vi "Get_alloys_list.vi"(7 "LabVIEW Web Service Request":refnum<class "Web Request.lvclass">) -> (2 "Alloys_group_arr":T1(array[cluster]))   [LabVIEW 2020]
uses:
  <vilib>/wsapi/Web Request.lvclass
  <vilib>/Utility/file.llb/Read Delimited Spreadsheet (string).vi
panel:
  # "Use the Web Service Request input terminal to call the VIs on the Web Services palette. Do not remove it from the connector pane unless you don't need access to the palette."
  # "Each additional control wired to the connector pane will be available as an input in the URL. To include an indicator in terminal-mode output (the default setting), it must also be wired to the connector pane."
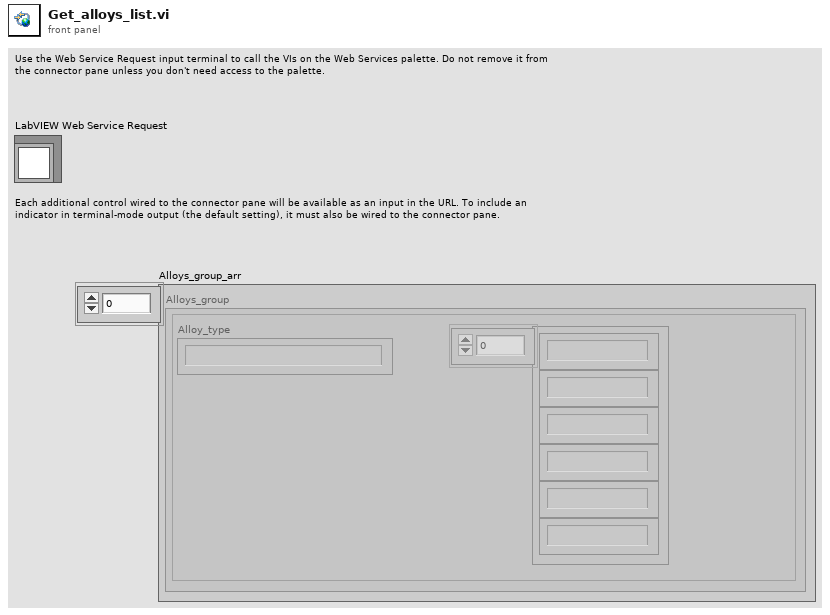
[diagram p1: front panel]
types:
  T1 = cluster{"Alloys":string[], "Alloy_type":string}[]
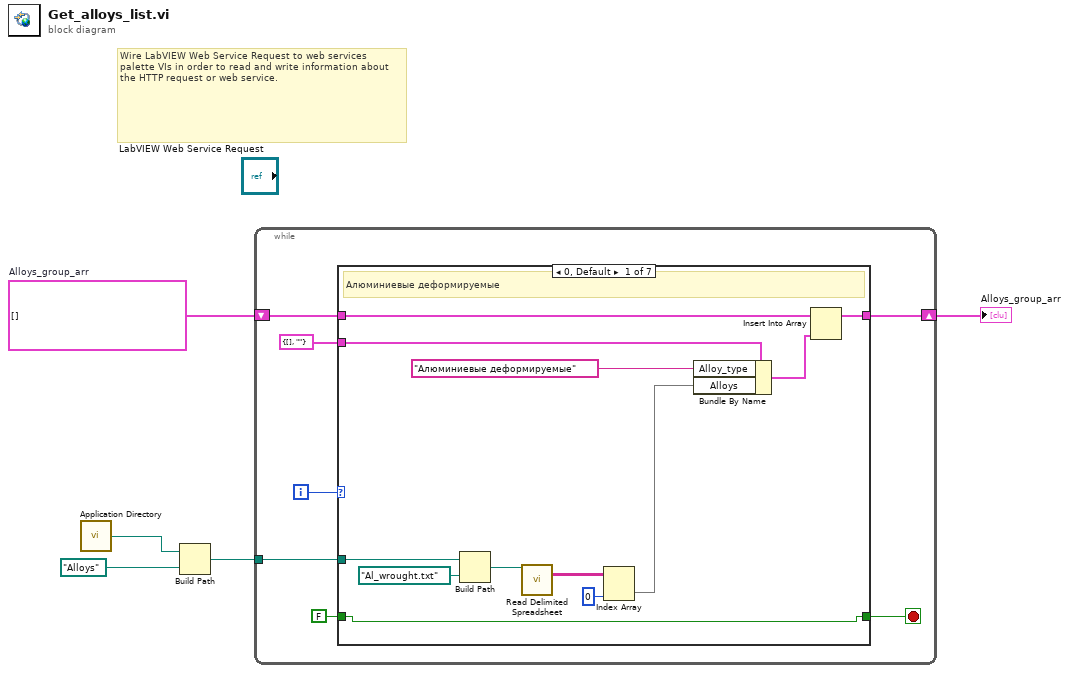
[diagram p0: block diagram]
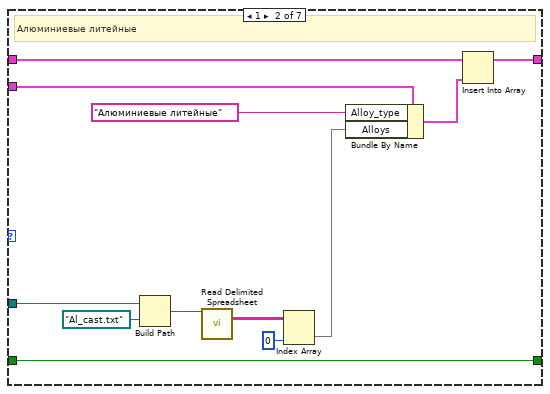
[diagram p2: hidden frame]
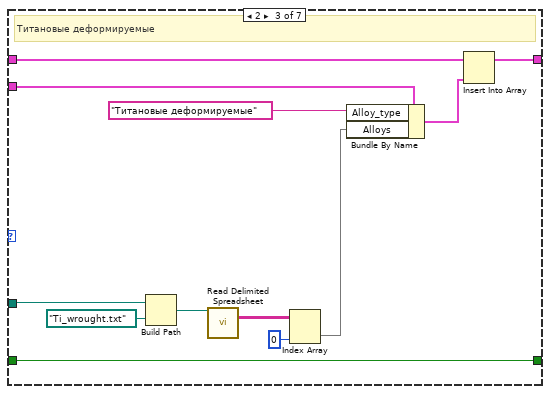
[diagram p3: hidden frame]
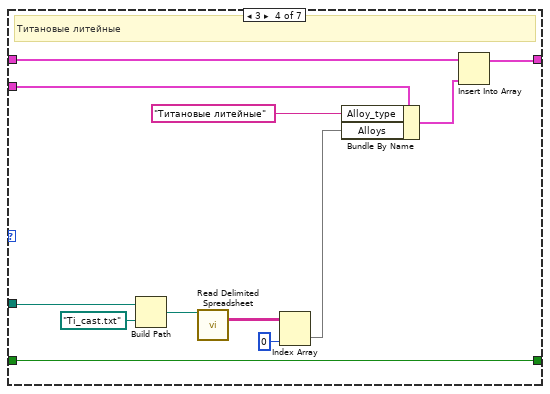
[diagram p4: hidden frame]
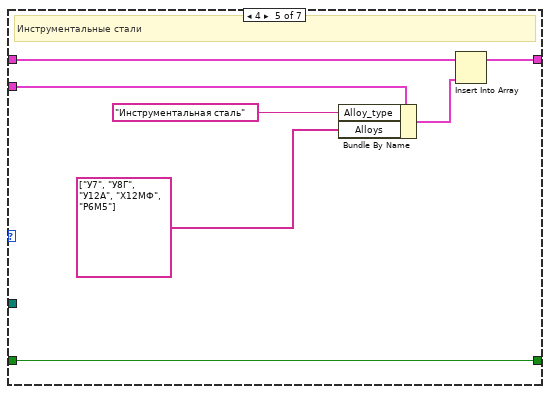
[diagram p5: hidden frame]
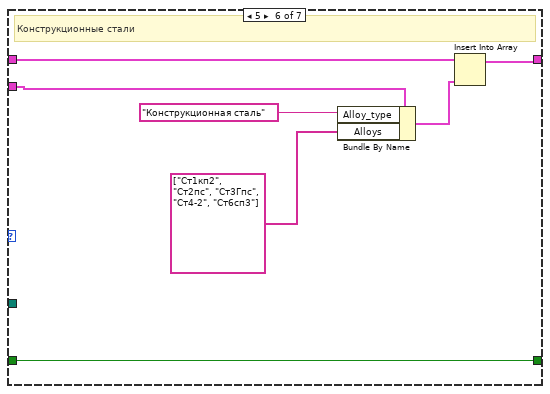
[diagram p6: hidden frame]
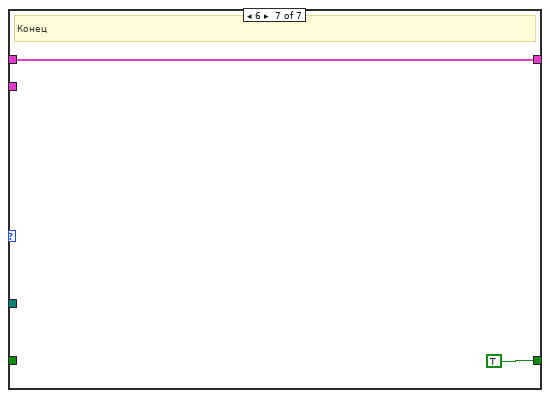
[diagram p7: hidden frame]
diagram:
  w5 = T1 []  # Alloys_group_arr
  # "Wire LabVIEW Web Service Request to web services palette VIs in order to read and write information about the HTTP request or web service."
  n1 = call <vilib>:"Application Directory.vi"() -> ("Application Directory"=w3:path)
  n2 = Build Path(base path=w3, name or relative path=path "Alloys") -> (appended path=w1:path)
  n3 = while {
    shift-right: [w10] -> w4
    shift-left: w5 -> [w9]
    tunnel: w1 -> [w7]
    i -> [w12]
    stop <- w11 stop-if-true
    n4 = case shown="0, Default" w12 {
      tunnel: [w17 w36 w48 w60 w67 w74 TRUE] -> w11
      tunnel: [w23 w34 w46 w58 w65 w71 w75] -> w10
      tunnel: w9 -> [w24 w33 w45 w57 w64 w72 w75]
      tunnel: cluster{"Alloys":string[], "Alloy_type":string} {"Alloys"=[], "Alloy_type"=""} ("new element/subarray") -> [w22 w32 w44 w56 w62 w69 _]
      tunnel: w7 -> [w20 w27 w38 w50 _ _ _]
      tunnel: FALSE -> [w17 w36 w48 w60 w67 w74 _]
      frame 0, Default {
        # "Алюминиевые деформируемые"
        n5 = Build Path(base path=w20, name or relative path=path "Al_wrought.txt") -> (appended path=w18:path)
        n6 = call-poly <vilib>:"Read Delimited Spreadsheet.vi"("file path (dialog if empty)"=w18) -> ("all rows"=w16:string[][])  [unwired: 9 in, 5 out]
        n7 = Index Array(array=w16, index (col)=0 ("disabled index (col)")) -> (element=w14:string[])  [unwired: 1 in]
        n8 = Bundle By Name(cluster=w22, "Alloy_type"="Алюминиевые деформируемые", "Alloys"=w14) -> (w21:cluster{"Alloys":string[], "Alloy_type":string})
        n9 = Insert Into Array(array=w24, new element=w21) -> (w23:T1)  [unwired: 1 in]
      }
      frame 1 {
        # "Алюминиевые литейные"
        n10 = Build Path(base path=w27, name or relative path=path "Al_cast.txt") -> (appended path=w30:path)
        n11 = call-poly <vilib>:"Read Delimited Spreadsheet.vi"("file path (dialog if empty)"=w30) -> ("all rows"=w29:string[][])  [unwired: 9 in, 5 out]
        n12 = Index Array(array=w29, index (col)=0 ("disabled index (col)")) -> (element=w26:string[])  [unwired: 1 in]
        n13 = Bundle By Name(cluster=w32, "Alloy_type"="Алюминиевые литейные", "Alloys"=w26) -> (w35:cluster{"Alloys":string[], "Alloy_type":string})
        n14 = Insert Into Array(array=w33, new element=w35) -> (w34:T1)  [unwired: 1 in]
      }
      frame 2 {
        # "Титановые деформируемые"
        n15 = Build Path(base path=w38, name or relative path=path "Ti_wrought.txt") -> (appended path=w41:path)
        n16 = call-poly <vilib>:"Read Delimited Spreadsheet.vi"("file path (dialog if empty)"=w41) -> ("all rows"=w40:string[][])  [unwired: 9 in, 5 out]
        n17 = Index Array(array=w40, index (col)=0 ("disabled index (col)")) -> (element=w37:string[])  [unwired: 1 in]
        n18 = Bundle By Name(cluster=w44, "Alloy_type"="Титановые деформируемые", "Alloys"=w37) -> (w47:cluster{"Alloys":string[], "Alloy_type":string})
        n19 = Insert Into Array(array=w45, new element=w47) -> (w46:T1)  [unwired: 1 in]
      }
      frame 3 {
        # "Титановые литейные"
        n20 = Build Path(base path=w50, name or relative path=path "Ti_cast.txt") -> (appended path=w54:path)
        n21 = call-poly <vilib>:"Read Delimited Spreadsheet.vi"("file path (dialog if empty)"=w54) -> ("all rows"=w53:string[][])  [unwired: 9 in, 5 out]
        n22 = Index Array(array=w53, index (col)=0 ("disabled index (col)")) -> (element=w49:string[])  [unwired: 1 in]
        n23 = Bundle By Name(cluster=w56, "Alloy_type"="Титановые литейные", "Alloys"=w49) -> (w59:cluster{"Alloys":string[], "Alloy_type":string})
        n24 = Insert Into Array(array=w57, new element=w59) -> (w58:T1)  [unwired: 1 in]
      }
      frame 4 {
        # "Инструментальные стали"
        n25 = Bundle By Name(cluster=w62, "Alloy_type"="Инструментальная сталь", "Alloys"=string[] ["У7", "У8Г", "У12А", "Х12МФ", "Р6М5"]) -> (w66:cluster{"Alloys":string[], "Alloy_type":string})
        n26 = Insert Into Array(array=w64, new element=w66) -> (w65:T1)  [unwired: 1 in]
      }
      frame 5 {
        # "Конструкционные стали"
        n27 = Bundle By Name(cluster=w69, "Alloy_type"="Конструкционная сталь", "Alloys"=string[] ["Ст1кп2", "Ст2пс", "Ст3Гпс", "Ст4-2", "Ст6сп3"]) -> (w73:cluster{"Alloys":string[], "Alloy_type":string})
        n28 = Insert Into Array(array=w72, new element=w73) -> (w71:T1)  [unwired: 1 in]
      }
      frame 6 {
        # "Конец"
      }
    }
  }
  "Alloys_group_arr" <- w4
